vi "Teleop.vi"(10 "Match Info":T1={"Autonomous Elapsed Seconds"=0.0, "TeleOp Elapsed Seconds"=23.585, "Disabled Elapsed Seconds"=1.934, "Visited Autonomous"=FALSE, "Visited TeleOp"=TRUE, "Visited Disabled"=TRUE, "Autonomous Settings"={"Autonomous Style"=enum."Independent", "VI Refnum"=refnum}}, 11 "Call Context":T2=enum."Stop") -> ()   [LabVIEW 2013]
doc: "This VI is called for each TeleOp packet received from the DS where the robot is not disabled. It is often used to read from the joysticks and update I/O or to update setpoints for timed control loops. It should complete and return within 20 milliseconds or it may miss DS packets."
uses:
  <vilib>/Rock Robotics/WPI/DriverStation/WPI_DriverStationDerivedRobotMode.ctl
  <vilib>/Rock Robotics/WPI/DriverStation/WPI_DriverStationMatch Info.ctl
  Robot Global Data.vi
  <vilib>/Rock Robotics/WPI/Joystick/WPI_JoystickGetSetRefNum.vi
panel:
  in  "Dead Zone(0 to 1)":dbl=0.25 format="%#_13g"
  in  "Left n^x":dbl=3.0 format="%#_13g"
  in  "Right n^x":dbl=1.25 format="%#_13g"
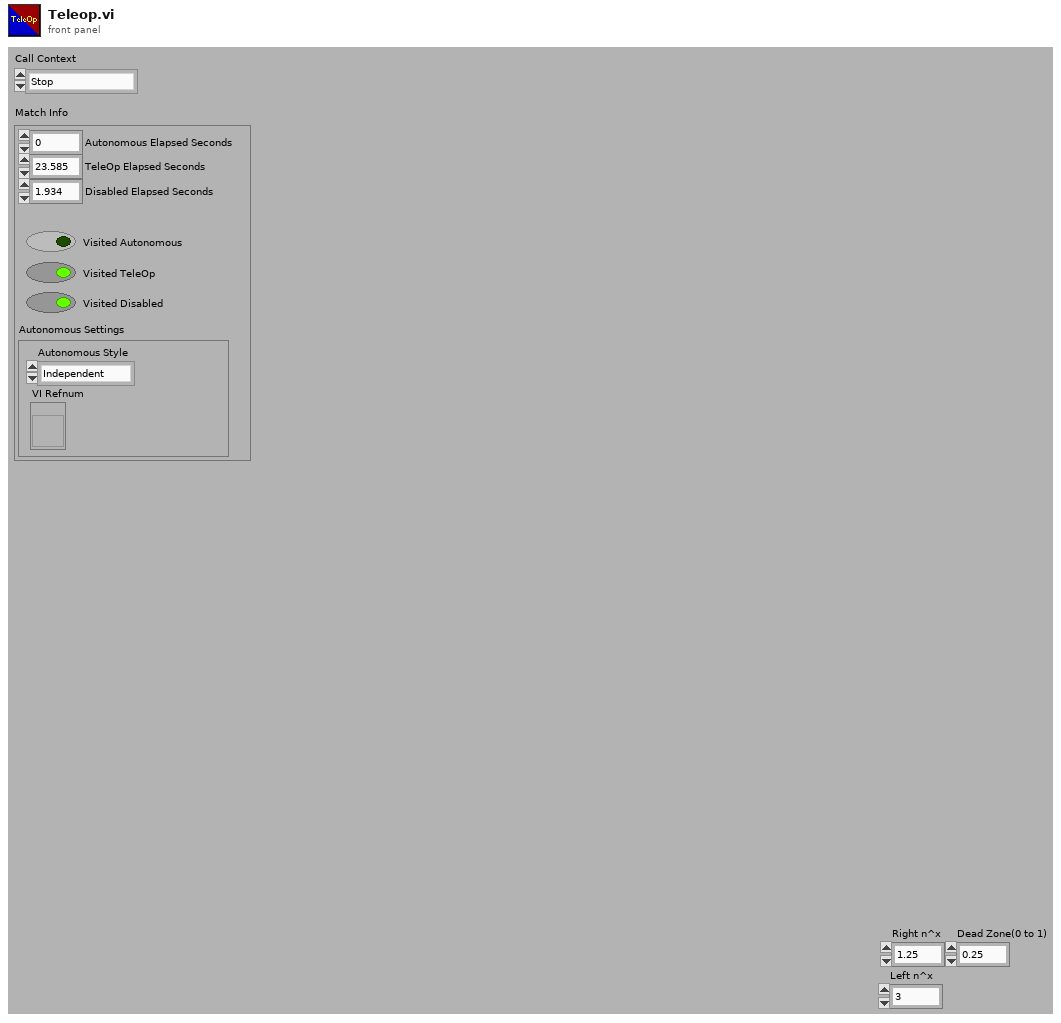
[diagram p1: front panel]
types:
  T1 = typedef "WPI_DriverStationMatch Info.ctl" = cluster{"Autonomous Elapsed Seconds":dbl, "TeleOp Elapsed Seconds":dbl, "Disabled Elapsed Seconds":dbl, "Visited Autonomous":bool, "Visited TeleOp":bool, "Visited Disabled":bool, "Autonomous Settings":cluster{"Autonomous Style":enum16{"Iterative", "Independent"}, "VI Refnum":refnum<vi>}}
  T2 = typedef "WPI_DriverStationDerivedRobotMode.ctl" = enum16{"Init", "Execute", "Stop"}
  T3 = enum16{"Linear", "Square  Root", "Square", "n^x"}
  T4 = typedef "WPI_JoystickDevRef.ctl" = cluster{"Device":T5}
  T5 = typedef "WPI_JoystickDeviceEnum.ctl" = enum16{"USB 1", "USB 2", "USB 3", "USB 4", "Kinect 1", "Kinect 2"}
  T6 = typedef "WPI_JoystickButtonState.ctl" = cluster{"Button 1":bool, "Button 2":bool, "Button 3":bool, "Button 4":bool, "Button 5":bool, "Button 6":bool, "Button 7":bool, "Button 8":bool, "Button 9":bool, "Button 10":bool, "Button 11":bool, "Button 12":bool}
  T7 = cluster{"axis 1 (x)":dbl, "axis 2 (y)":dbl, "axis 3 (throttle)":dbl, "axis 4":dbl, "axis 5":dbl, "axis 6":dbl}
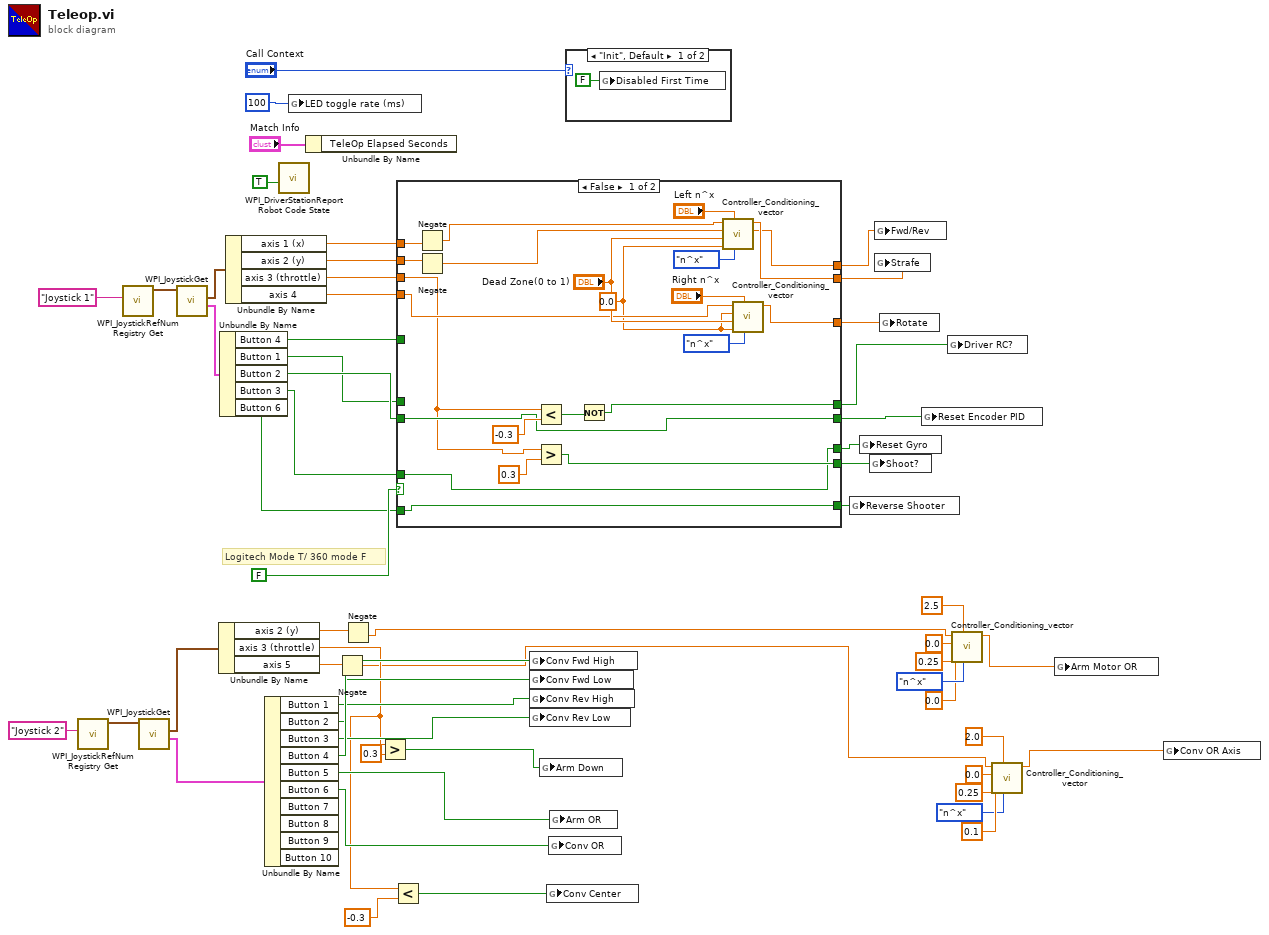
[diagram p0: block diagram]
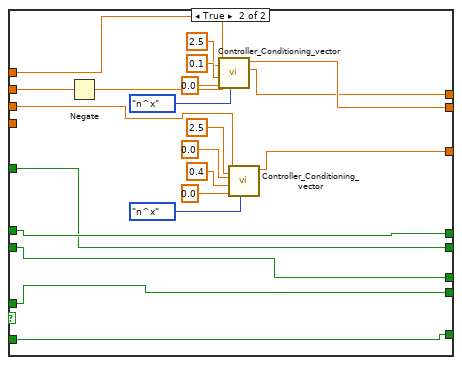
[diagram p2: hidden frame]
diagram:
  # "Logitech Mode T/ 360 mode F"
  n1 = call <vilib>:"WPI_JoystickRefNum Registry Get.vi"("refnum name"="Joystick 2") -> ("JoystickDevRef"=w50:T4)  [unwired: 1 in, 9 out]
  n2 = call <vilib>:"WPI_JoystickRefNum Registry Get.vi"("refnum name"="Joystick 1") -> ("JoystickDevRef"=w55:T4)  [unwired: 1 in, 9 out]
  n3 = call <vilib>:"WPI_JoystickGet.vi"("JoystickDevRef"=w50) -> ("Buttons"=w35:T6, "Axes"=w49:T7)  [unwired: 1 in, 4 out]
  n4 = call <vilib>:"WPI_JoystickGet.vi"("JoystickDevRef"=w55) -> ("Buttons"=w48:T6, "Axes"=w52:T7)  [unwired: 1 in, 4 out]
  n5 = Unbundle By Name(w49) -> ("axis 2 (y)"=w24:dbl, "axis 3 (throttle)"=w20:dbl, "axis 5"=w21:dbl)
  n6 = Unbundle By Name(w48) -> ("Button 4"=w31:bool, "Button 1"=w36:bool, "Button 2"=w43:bool, "Button 3"=w33:bool, "Button 6"=w16:bool)
  n7 = Unbundle By Name(w52) -> ("axis 1 (x)"=w46:dbl, "axis 2 (y)"=w45:dbl, "axis 3 (throttle)"=w42:dbl, "axis 4"=w44:dbl)
  n8 = Unbundle By Name(w35) -> ("Button 1"=w29:bool, "Button 2"=w28:bool, "Button 3"=w27:bool, "Button 4"=w30:bool, "Button 5"=w23:bool, "Button 6"=w22:bool)  [unwired: 4 out]
  n9 = call <vilib>:"WPI_DriverStationReport Robot Code State.vi"("TeleOp"=TRUE ("Autonomous")) -> ()  [unwired: 10 in, 1 out]
  n10 = global write "Robot Global Data.vi" "LED toggle rate (ms)"(u32 100 ("LED ms toggle rate")) -> ()
  n11 = Unbundle By Name("Match Info") -> ()  [unwired: 1 out]
  n12 = Negate(x=w21) -> (-x=w2:dbl)
  n13 = Negate(x=w24) -> (-x=w12:dbl)
  n14 = Greater?(x=w20, y=0.3) -> (0:w25:bool)
  n15 = Less?(x=w20, y=-0.3) -> (x < y?=w18:bool)
  n16 = case shown="False" FALSE {
    tunnel: w46 -> [w74 w96]
    tunnel: w45 -> [w73 w101]
    tunnel: w44 -> [w64 _]
    tunnel: w43 -> [w79 w99]
    tunnel: w42 -> [w59 w84]
    tunnel: [w60 w89] -> w17
    tunnel: [w61 w90] -> w40
    tunnel: [w75 w100] -> w39
    tunnel: [w63 w88] -> w38
    tunnel: [w79 w98] -> w37
    tunnel: w36 -> [_ w100]
    tunnel: w33 -> [w72 w97]
    tunnel: [w77 w97] -> w34
    tunnel: [w72 w99] -> w32
    tunnel: w31 -> [_ w98]
    tunnel: w16 -> [w58 w81]
    tunnel: [w58 w81] -> w15
    frame False {
      w62 = 0.0 ("Y(-1 to 1)")
      n17 = Negate(x=w74) -> (-x=w66:dbl)
      n18 = Negate(x=w73) -> (-x=w65:dbl)
      n19 = Less?(x=w59, y=-0.3) -> (x < y?=w76:bool)
      n20 = Greater?(x=w59, y=0.3) -> (0:w77:bool)
      n21 = Not(x=w76) -> (.not. x?=w75:bool)
      n22 = call "Controller_Conditioning_vector.vi"("Enum"=T3."n^x", "n^x(Unbounded)"="Left n^x", "Min Output(0 to 1)"=w62, "Dead Zone(0 to 1)"="Dead Zone(0 to 1)", "Y(-1 to 1)"=w65, "X(-1 to 1)"=w66) -> ("Y"=w60:dbl, "X"=w61:dbl)  [unwired: 1 in, 2 out]
      n23 = call "Controller_Conditioning_vector.vi"("Enum"=T3."n^x", "n^x(Unbounded)"="Right n^x", "Min Output(0 to 1)"=w62, "Dead Zone(0 to 1)"="Dead Zone(0 to 1)", "Y(-1 to 1)"=w62, "X(-1 to 1)"=w64) -> ("X"=w63:dbl)  [unwired: 1 in, 3 out]
    }
    frame True {
      n24 = Negate(x=w101) -> (-x=w95:dbl)
      n25 = call "Controller_Conditioning_vector.vi"("Enum"=T3."n^x", "n^x(Unbounded)"=2.5, "Min Output(0 to 1)"=0.0, "Dead Zone(0 to 1)"=0.1, "Y(-1 to 1)"=w95, "X(-1 to 1)"=w96) -> ("Y"=w89:dbl, "X"=w90:dbl)  [unwired: 1 in, 2 out]
      n26 = call "Controller_Conditioning_vector.vi"("Enum"=T3."n^x", "n^x(Unbounded)"=2.5, "Min Output(0 to 1)"=0.0, "Dead Zone(0 to 1)"=0.4, "Y(-1 to 1)"=0.0, "X(-1 to 1)"=w84) -> ("X"=w88:dbl)  [unwired: 1 in, 3 out]
    }
  }
  n27 = global write "Robot Global Data.vi" "Conv Fwd High"(w30) -> ()
  n28 = global write "Robot Global Data.vi" "Conv Fwd Low"(w28) -> ()
  n29 = global write "Robot Global Data.vi" "Conv Rev High"(w29) -> ()
  n30 = global write "Robot Global Data.vi" "Conv Rev Low"(w27) -> ()
  n31 = global write "Robot Global Data.vi" "Arm Down"(w25) -> ()
  n32 = global write "Robot Global Data.vi" "Conv Center"(w18) -> ()
  n33 = global write "Robot Global Data.vi" "Conv OR"(w22) -> ()
  n34 = global write "Robot Global Data.vi" "Arm OR"(w23) -> ()
  n35 = case shown="\"Init\", Default" "Call Context" {
    frame "Init", Default {
      n36 = global write "Robot Global Data.vi" "Disabled First Time"(FALSE ("Disabled First Time")) -> ()
    }
    frame "Execute" {
    }
  }
  n37 = global write "Robot Global Data.vi" "Reverse Shooter"(w15) -> ()
  n38 = global write "Robot Global Data.vi" "Reset Gyro"(w32) -> ()
  n39 = global write "Robot Global Data.vi" "Shoot?"(w34) -> ()
  n40 = global write "Robot Global Data.vi" "Fwd/Rev"(w17) -> ()
  n41 = global write "Robot Global Data.vi" "Strafe"(w40) -> ()
  n42 = global write "Robot Global Data.vi" "Rotate"(w38) -> ()
  n43 = global write "Robot Global Data.vi" "Reset Encoder PID"(w37) -> ()
  n44 = global write "Robot Global Data.vi" "Driver RC?"(w39) -> ()
  n45 = call "Controller_Conditioning_vector.vi"("Enum"=T3."n^x", "n^x(Unbounded)"=2.5, "Min Output(0 to 1)"=0.0, "Dead Zone(0 to 1)"=0.25, "Y(-1 to 1)"=0.0, "X(-1 to 1)"=w12) -> ("X"=w14:dbl)  [unwired: 1 in, 3 out]
  n46 = call "Controller_Conditioning_vector.vi"("Enum"=T3."n^x", "n^x(Unbounded)"=2.0, "Min Output(0 to 1)"=0.1, "Dead Zone(0 to 1)"=0.25, "Y(-1 to 1)"=0.0, "X(-1 to 1)"=w2) -> ("X"=w1:dbl)  [unwired: 1 in, 3 out]
  n47 = global write "Robot Global Data.vi" "Arm Motor OR"(w14) -> ()
  n48 = global write "Robot Global Data.vi" "Conv OR Axis"(w1) -> ()
